vi "Auto Shoot Cube Command.vi"(8 "Command Info In":T2, 11 "Shoot Cube Parameters":cluster{"Shot Preset":T1}) -> (0 "Command Info Out":T2)   [LabVIEW 2020]
doc: "This template is useful for immediate subsystem actions that do not need deadband filtering\n\nBe sure to right-click and select New from Template and save with a new command name."
uses:
  <vilib>/Rock Robotics/WPI/Framework/Command Status Info.ctl
  <vilib>/Rock Robotics/WPI/Framework/Completion Status.ctl
  <vilib>/Rock Robotics/WPI/Framework/Completion Notifier.ctl
  Implementation/Typedefs/Cube Shooting Presets.ctl
  intake sub/Implementation/Typedef/intake typedef.ctl
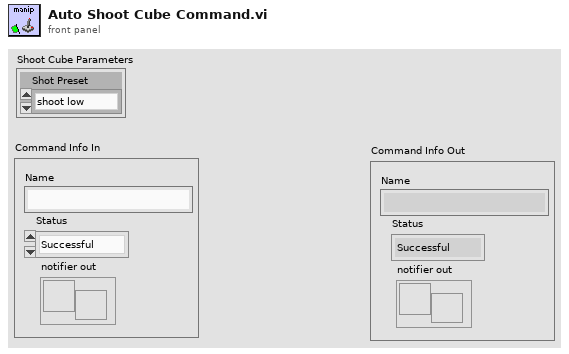
[diagram p1: front panel]
types:
  T1 = typedef "Cube Shooting Presets.ctl" = enum16{"shoot low", "shoot mid", "shoot high"}
  T2 = typedef "Command Status Info.ctl" = cluster{"Name":string, "Status":T3, "notifier out":T4}
  T3 = typedef "Completion Status.ctl" = enum16{"Successful", "Aborted", "Incomplete"}
  T4 = typedef "Completion Notifier.ctl" = refnum<notifier>
  T5 = typedef "intake typedef.ctl" = enum16{"Intake Cone Sideways", "Intake Cone Upright", "Intake Cube", "Outtake/Score", "Shoot"}
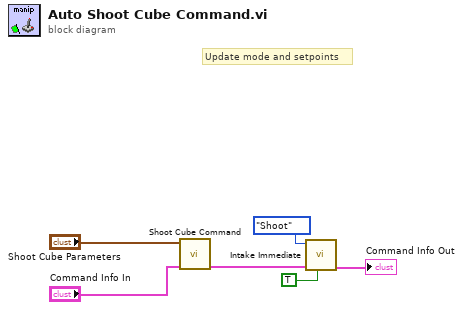
[diagram p0: block diagram]
diagram:
  # "Update mode and setpoints"
  n1 = call "Shoot Cube Command.vi"("Command Info In"="Command Info In", "Shoot Cube Parameters"="Shoot Cube Parameters") -> ("Command Info Out"=w1:T2)  [unwired: 9 in]
  n2 = call "Intake Immediate.vi"("Wait for Manipulator"=TRUE, "Command Info In"=w1, "intake modes"=intake_typedef."Shoot") -> ("Command Info Out"=→"Command Info Out":T2)  [unwired: 8 in]
